vi "MHL Cases.vi"(8 "error in":errorcluster, 11 "Base Hardware in":refnum<class "Base Hardware.lvclass">) -> (0 "error out":errorcluster, 3 "Base Hardware out":refnum<class "Base Hardware.lvclass">)   [LabVIEW 2023, in "Abstract Hardware.lvlib" / "Base Hardware.lvclass"]
doc: "The base class Message Handling Loop cases of a Worker's QMH."
uses:
  Base Hardware.lvclass
  C:/Program Files/National Instruments/LabVIEW 2023/vi.lib/addons/_Workers/Library/Classes/Worker/Worker.lvclass
  <vilib>/addons/_Workers/Library/Classes/Worker/Worker.lvclass/Worker.ctl
  <vilib>/addons/_Workers/Library/Classes/Message/Message.lvclass/Message.ctl
  Initialization Data.ctl
  Response Cases.ctl
  <vilib>/addons/_Workers/Library/Case Label.ctl
  Settings.ctl
  Base Hardware.lvclass/Base Hardware.ctl
  rql_Read-Write Error.ctl
  rqp_Init.ctl
  rqp_Close.ctl
  rqp_Write.ctl
  rqp_Read.ctl
  rqp_REINIT.ctl
  rqp_Edit Polling.ctl
  rwr_Init With Reply.ctl
  rwr_Init With Reply Reply.ctl
  rqp_Update Internal Data.ctl
  rqp_Show Panel.ctl
  <vilib>/addons/_Workers/Library/Classes/Message/Priority.ctl
  <vilib>/Utility/error.llb/Error Cluster From Error Code.vi
  <vilib>/ErrorRing/Error Ring.xnode
  <vilib>/addons/_Workers/Library/Classes/Message Queue/Message Queue.lvclass
  <vilib>/addons/_Workers/Library/Classes/Worker/Worker.lvclass
  <vilib>/addons/_Workers/Library/Classes/Message/Message.lvclass
  Message Pump/Message Pump.lvclass
  <vilib>/addons/_Workers/Library/Workers.lvlib
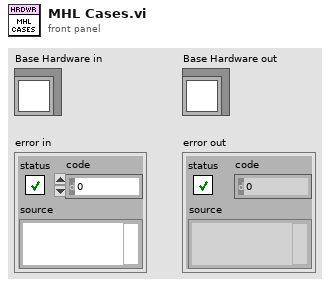
[diagram p1: front panel]
types:
  T1 = typedef "Workers.lvlib/Case Label.ctl" = string
  T2 = typedef "Abstract Hardware.lvlib/Base Hardware.lvclass/Initialization Data.ctl" = cluster{"Response Cases":T3, "Settings":T4}
  T3 = typedef "Abstract Hardware.lvlib/Base Hardware.lvclass/Response Cases.ctl" = cluster{"Placeholder - Can be deleted":string, "Get Data":T1, "Get Init Result":T1}
  T4 = typedef "Abstract Hardware.lvlib/Base Hardware.lvclass/Settings.ctl" = cluster{"Polling Period, ms":i64}
  T5 = typedef "Abstract Hardware.lvlib/Base Hardware.lvclass/rql_Read-Write Error.ctl" = cluster{"String":string}
  T6 = typedef "Abstract Hardware.lvlib/Base Hardware.lvclass/rqp_Init.ctl" = variant
  T7 = typedef "Abstract Hardware.lvlib/Base Hardware.lvclass/rqp_Close.ctl" = cluster{"String":string}
  T8 = typedef "Abstract Hardware.lvlib/Base Hardware.lvclass/rqp_Write.ctl" = variant
  T9 = typedef "Abstract Hardware.lvlib/Base Hardware.lvclass/rqp_Read.ctl" = cluster{"String":string}
  T10 = typedef "Abstract Hardware.lvlib/Base Hardware.lvclass/rqp_REINIT.ctl" = variant
  T11 = typedef "Abstract Hardware.lvlib/Base Hardware.lvclass/rqp_Edit Polling.ctl" = i64
  T12 = typedef "Abstract Hardware.lvlib/Base Hardware.lvclass/rwr_Init With Reply Reply.ctl" = cluster{"String":string}
  T13 = typedef "Abstract Hardware.lvlib/Base Hardware.lvclass/rwr_Init With Reply.ctl" = cluster{"String":string}
  T14 = typedef "Abstract Hardware.lvlib/Base Hardware.lvclass/rqp_Update Internal Data.ctl" = variant
  T15 = typedef "Abstract Hardware.lvlib/Base Hardware.lvclass/rqp_Show Panel.ctl" = cluster{"String":string}
  T16 = typedef "Workers.lvlib/Message.lvclass/Priority.ctl" = enum16{"Low", "Normal", "High"}
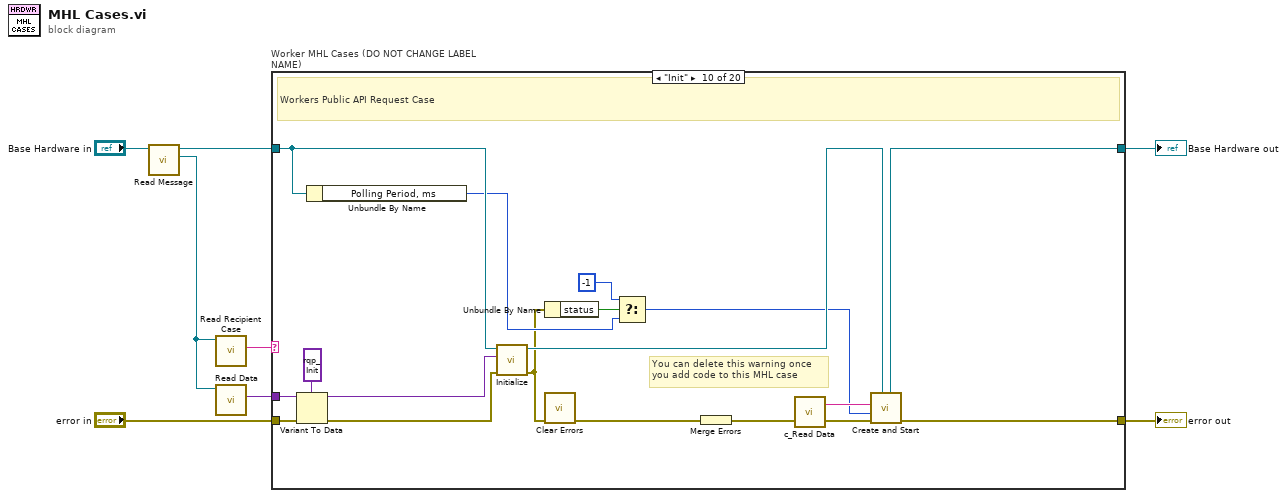
[diagram p0: block diagram]
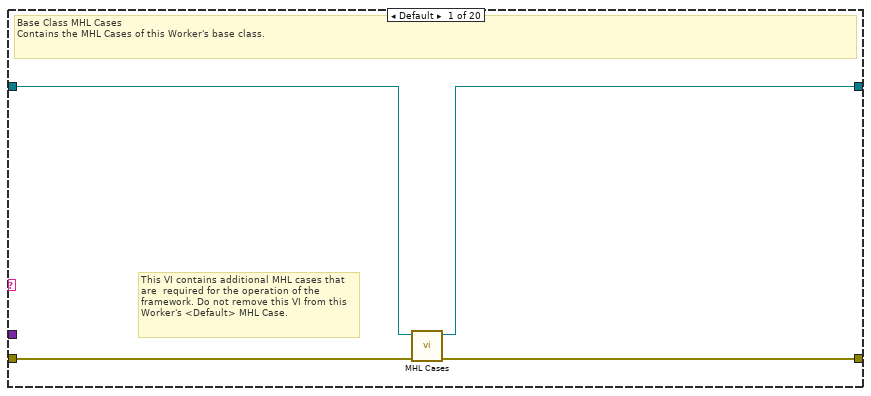
[diagram p2: hidden frame]
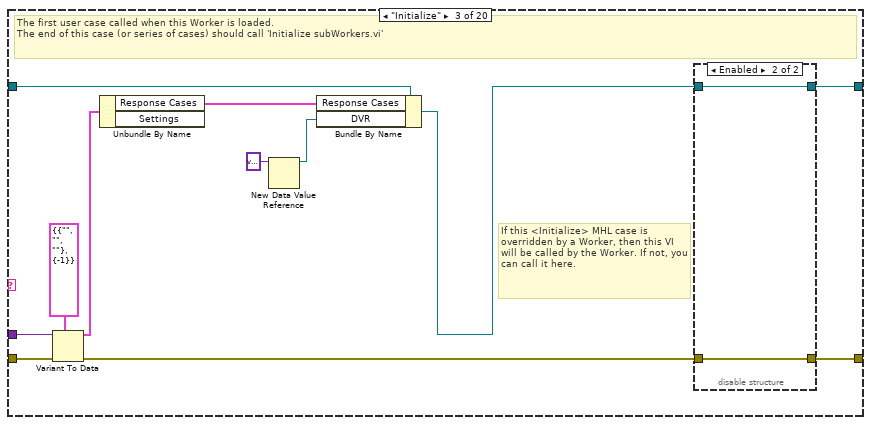
[diagram p4: hidden frame]
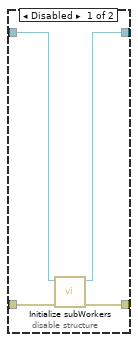
[diagram p5: hidden frame]
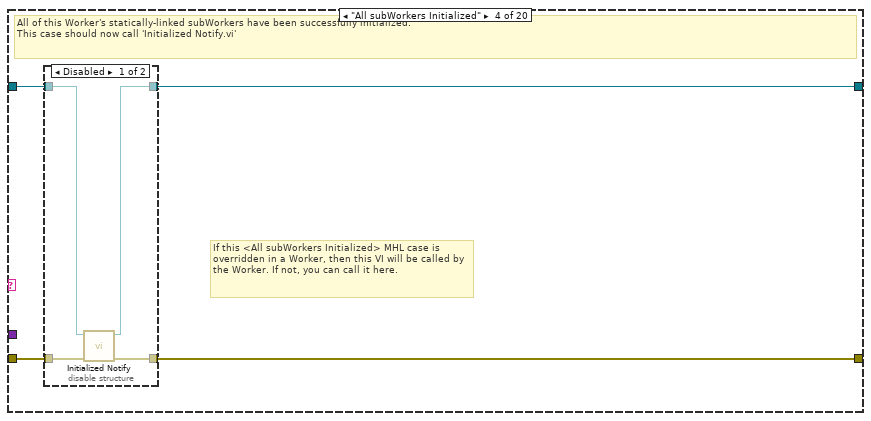
[diagram p6: hidden frame]
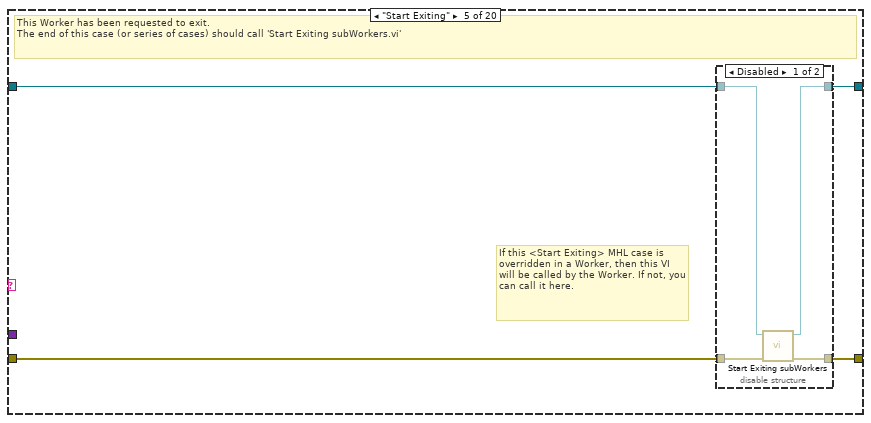
[diagram p8: hidden frame]
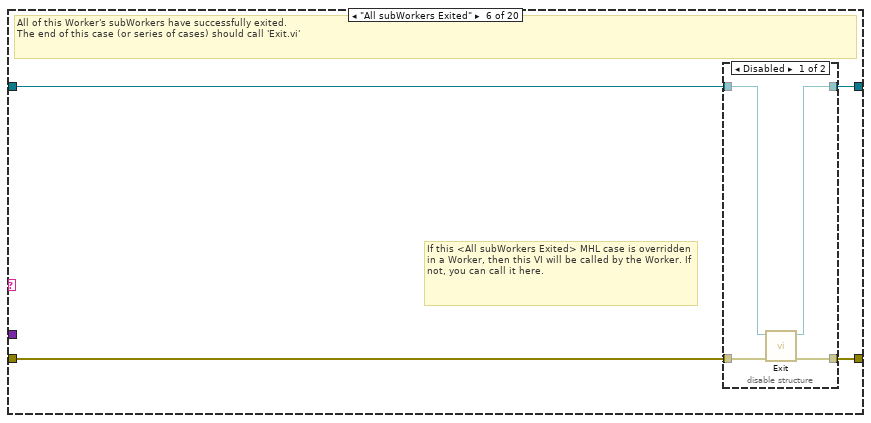
[diagram p10: hidden frame]
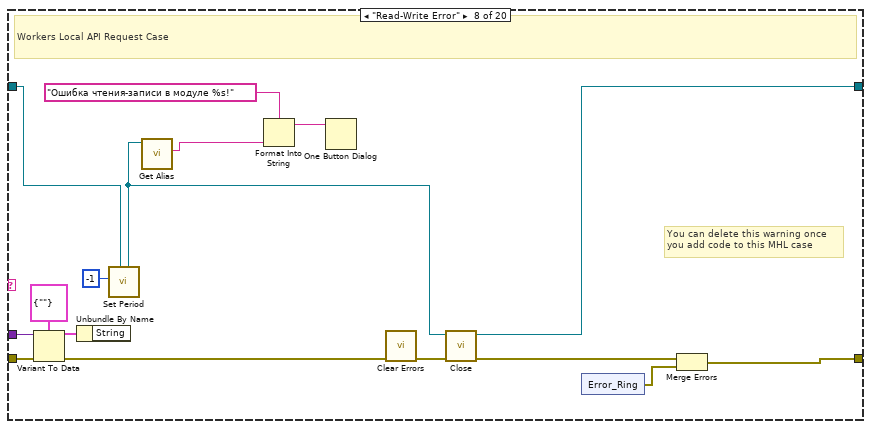
[diagram p13: hidden frame]
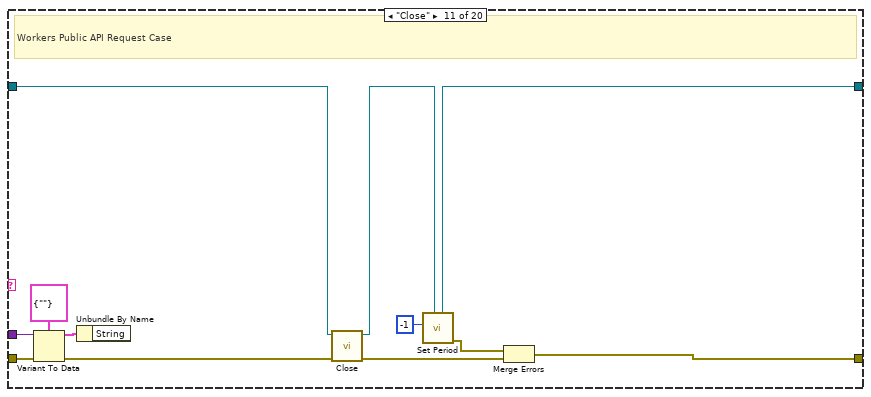
[diagram p15: hidden frame]
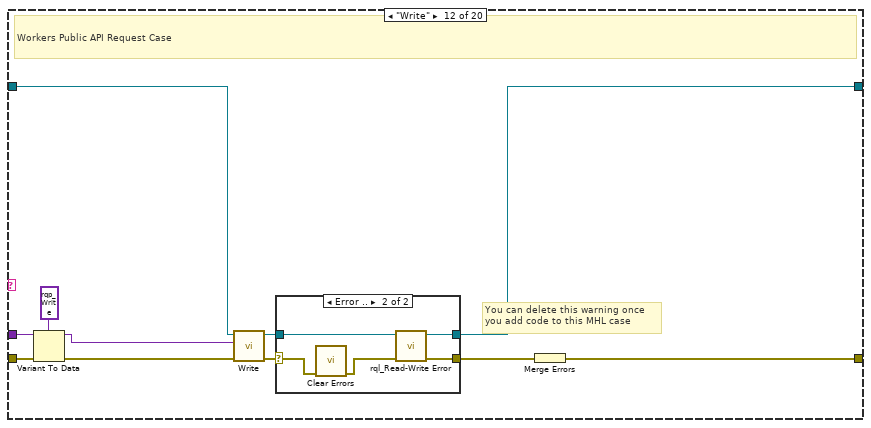
[diagram p16: hidden frame]
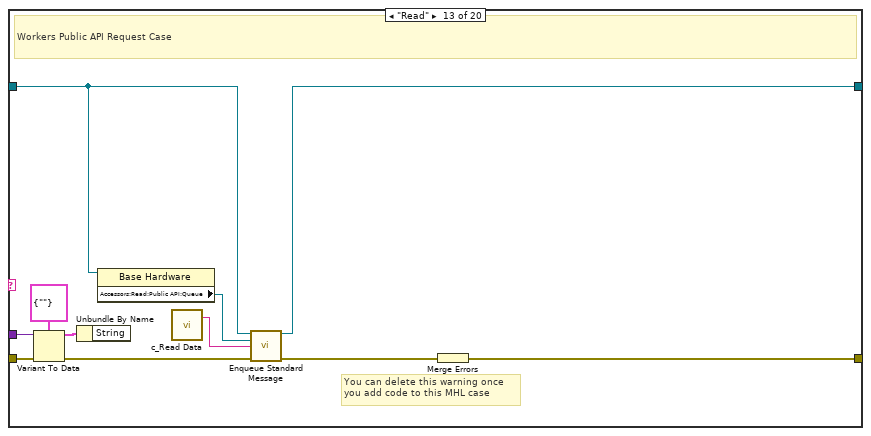
[diagram p18: hidden frame]
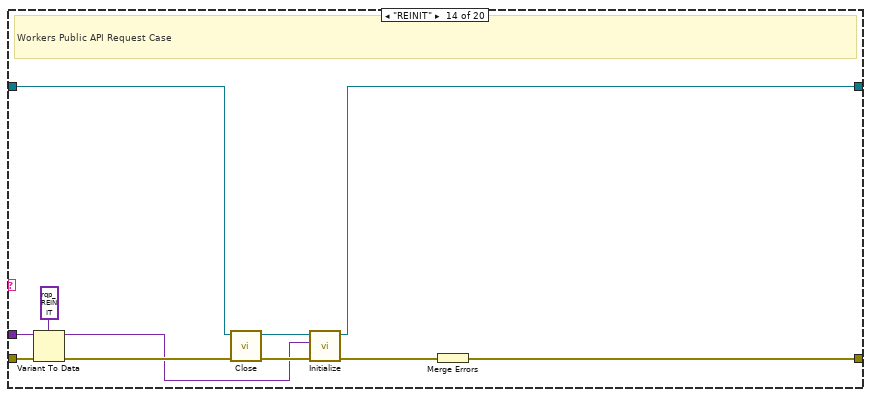
[diagram p19: hidden frame]
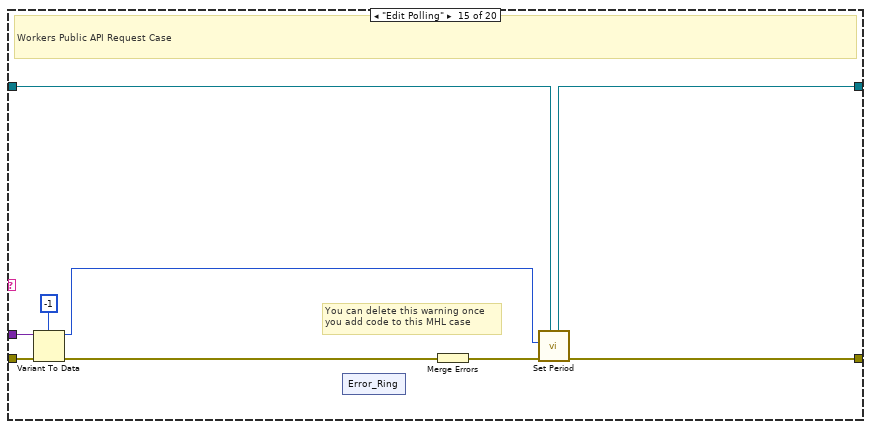
[diagram p20: hidden frame]
diagram:
  n1 = call <vilib>:"Read Message.vi"("Worker"="Base Hardware in") -> ("Message"=w3:refnum<class "Message.lvclass">, "dup Worker out"=w8:refnum<class "Base Hardware.lvclass">)  [unwired: 9 in]
  n2 = call <vilib>:"Read Recipient Case.vi"("Message"=w3) -> ("Recipient Case"=w7:T1)  [unwired: 9 in, 1 out]
  n3 = call <vilib>:"Read Data.vi"("Message"=w3) -> ("Data"=w1:variant)  [unwired: 9 in, 1 out]
  n4 = case "Worker MHL Cases (DO NOT CHANGE LABEL NAME)" shown="\"Init\"" w7 {
    tunnel: [w12 w14 w21 w33 w44 w55 w64 w76 w87 w88 w112 w121 w141 w153 w159 w176 w188 w205 w216 w219] -> w6
    tunnel: [w11 w13 w20 w35 w45 w53 w63 w71 w86 w100 w106 w119 w140 w146 w160 w175 w193 w200 w215 w220] -> w5
    tunnel: "error in" -> [w10 w14 w26 w34 w43 w56 w64 w80 w87 w104 w116 w127 w145 w156 w165 w181 w192 w209 w216 w221]
    tunnel: w8 -> [w9 w13 w17 w36 w46 w54 w63 w70 w86 w96 w109 w124 w136 w151 w161 w174 w193 w203 w215 w218]
    tunnel: w1 -> [_ _ w25 _ _ _ _ w78 _ w102 w114 w125 w143 w154 w162 w178 w189 w207 _ _]
    frame Default {
      # "This VI contains additional MHL cases that are  required for the operation of the framework. Do not remove this VI from this Worker's <Default> MHL Case."
      # "Base Class MHL Cases\nContains the MHL Cases of this Worker's base class."
      n5 = call-parent "MHL Cases.vi"("error in"=w10, "Worker in"=w9) -> ("error out"=w12:errorcluster, "Worker out"=w11:refnum<class "Base Hardware.lvclass">)  [unwired: 8 in]
    }
    frame "------------ FRAMEWORK CASES -----------" {
      # "Start of Workers Framework Cases"
    }
    frame "Initialize" {
      # "If this <Initialize> MHL case is overridden by a Worker, then this VI will be called by the Worker. If not, you can call it here."
      # "The first user case called when this Worker is loaded.\nThe end of this case (or series of cases) should call 'Initialize subWorkers.vi'"
      n6 = Variant To Data(error in=w26, type=T2 {"Response Cases"={"Placeholder - Can be deleted"="", "Get Data"="", "Get Init Result"=""}, "Settings"={"Polling Period, ms"=-1}} ("Initialization Data"), Variant=w25) -> (data=w24:T2, error out=w15:errorcluster)
      n7 = Unbundle By Name(w24) -> ("Response Cases"=w23:T3)  [unwired: 1 out]
      n8 = New Data Value Reference(data value=variant) -> (data value reference=w18:refnum<data-value>)  [unwired: 1 in, 1 out]
      n9 = Bundle By Name(cluster=w17, "Response Cases"=w23, "DVR"=w18) -> (w16:refnum<class "Base Hardware.lvclass">)
      n10 = disable-structure shown="Enabled" {
        disable-tunnel: w15 -> [w30 w31]
        disable-tunnel: [w29 w31] -> w21
        disable-tunnel: w16 -> [w28 w32]
        disable-tunnel: [w27 w32] -> w20
        frame Disabled {
          n11 = call-dynamic "Initialize subWorkers.vi"("error in"=w30, "Base Hardware"=w28) -> ("error out"=w29:errorcluster, "dup Base Hardware out"=w27:refnum<class "Base Hardware.lvclass">)  [unwired: 8 in]
        }
        frame Enabled {
        }
      }
    }
    frame "All subWorkers Initialized" {
      # "If this <All subWorkers Initialized> MHL case is overridden in a Worker, then this VI will be called by the Worker. If not, you can call it here."
      # "All of this Worker's statically-linked subWorkers have been successfully initialized.\nThis case should now call 'Initialized Notify.vi'"
      n12 = disable-structure shown="Disabled" {
        disable-tunnel: w36 -> [w40 w42]
        disable-tunnel: [w39 w42] -> w35
        disable-tunnel: w34 -> [w38 w41]
        disable-tunnel: [w37 w41] -> w33
        frame Disabled {
          n13 = call-dynamic "Initialized Notify.vi"("error in"=w38, "Worker"=w40) -> ("error out"=w37:errorcluster, "dup Worker out"=w39:refnum<class "Base Hardware.lvclass">)  [unwired: 8 in]
        }
        frame Enabled {
        }
      }
    }
    frame "Start Exiting" {
      # "If this <Start Exiting> MHL case is overridden in a Worker, then this VI will be called by the Worker. If not, you can call it here."
      # "This Worker has been requested to exit. \nThe end of this case (or series of cases) should call 'Start Exiting subWorkers.vi'"
      n14 = disable-structure shown="Disabled" {
        disable-tunnel: w46 -> [w50 w52]
        disable-tunnel: [w49 w52] -> w45
        disable-tunnel: [w48 w51] -> w44
        disable-tunnel: w43 -> [w47 w51]
        frame Disabled {
          n15 = call-dynamic "Start Exiting subWorkers.vi"("error_in"=w47, "Worker"=w50) -> ("error out"=w48:errorcluster, "dup Worker out"=w49:refnum<class "Base Hardware.lvclass">)  [unwired: 8 in]
        }
        frame Enabled {
        }
      }
    }
    frame "All subWorkers Exited" {
      # "If this <All subWorkers Exited> MHL case is overridden in a Worker, then this VI will be called by the Worker. If not, you can call it here."
      # "All of this Worker's subWorkers have successfully exited. \nThe end of this case (or series of cases) should call 'Exit.vi'"
      n16 = disable-structure shown="Disabled" {
        disable-tunnel: w56 -> [w60 w61]
        disable-tunnel: [w59 w61] -> w55
        disable-tunnel: w54 -> [w58 w62]
        disable-tunnel: [w57 w62] -> w53
        frame Disabled {
          n17 = call-dynamic "Exit.vi"("error_in"=w60, "Worker"=w58) -> ("error out"=w59:errorcluster, "dup Worker out"=w57:refnum<class "Base Hardware.lvclass">)  [unwired: 8 in]
        }
        frame Enabled {
        }
      }
    }
    frame "------------- LOCAL API CASES -------------" {
      # "Start of Workers Local API Cases"
    }
    frame "Read-Write Error" {
      # "You can delete this warning once\nyou add code to this MHL case"
      # "Workers Local API Request Case"
      n18 = Variant To Data(error in=w80, type=T5 {"String"=""} ("Data"), Variant=w78) -> (data=w77:T5, error out=w66:errorcluster)
      n19 = Unbundle By Name(w77) -> ()  [unwired: 1 out]
      n20 = call "Set Period.vi"("Caller"=w70, "Period (ms)"=-1) -> ("dup Caller out"=w69:refnum<class "Base Hardware.lvclass">)  [unwired: 8 in, 1 out]
      n21 = call-dynamic "Get Alias.vi"("Worker_"=w69) -> ("Alias"=w67:string)  [unwired: 8 in, 2 out]
      n22 = Format Into String(format string="Ошибка чтения-записи в модуле %s!", w67) -> (resulting string=w65:string)  [unwired: 2 in, 1 out]
      n23 = One Button Dialog(message=w65) -> ()  [unwired: 1 in, 1 out]
      n24 = call <vilib>:"Clear Errors.vi"("error in (no error)"=w66) -> ("error out"=w73:errorcluster)  [unwired: 5 in, 1 out]
      n25 = call-dynamic "Close.vi"("error in (no error)"=w73, "Base Hardware in"=w69) -> ("error out"=w72:errorcluster, "Base Hardware out"=w71:refnum<class "Base Hardware.lvclass">)  [unwired: 8 in]
      n26 = xnode ("Error_Ring")() -> ("error out"=w75:errorcluster)
      n27 = Merge Errors(w72, w75) -> (w76:errorcluster)
    }
    frame "------------- PUBLIC API CASES -------------" {
      # "Start of Workers Public API Cases"
    }
    frame "Init" {
      # "You can delete this warning once\nyou add code to this MHL case"
      # "Workers Public API Request Case"
      n28 = Variant To Data(error in=w104, type=T6 variant(string "") ("Data"), Variant=w102) -> (data=w95:T6, error out=w97:errorcluster)
      n29 = Unbundle By Name(w96) -> ("Polling Period, ms"=w93:i64)
      n30 = call-dynamic "Initialize.vi"("error in (no error)"=w97, "Settings"=w95, "Base Hardware in"=w96) -> ("error out"=w89:errorcluster, "Base Hardware out"=w98:refnum<class "Base Hardware.lvclass">)  [unwired: 7 in]
      n31 = Unbundle By Name(w89) -> ("status"=w94:bool)
      n32 = call <vilib>:"Clear Errors.vi"("error in (no error)"=w89) -> ("error out"=w90:errorcluster)  [unwired: 5 in, 1 out]
      n33 = Select(t=i64 -1, s=w94, f=w93) -> (s? t:f=w91:i64)
      n34 = Merge Errors(w90) -> (w99:errorcluster)
      n35 = call "c_Read Data.vi"() -> ("Case Label"=w101:T1)  [unwired: 1 in]
      n36 = call "Create and Start.vi"("Caller"=w98, "error in (no error)"=w99, "Period (ms)"=w91, "Time Elapsed Response Case (Case Label)"=w101) -> ("error out"=w88:errorcluster, "dup Caller out"=w100:refnum<class "Base Hardware.lvclass">)  [unwired: 5 in, 1 out]
    }
    frame "Close" {
      # "Workers Public API Request Case"
      n37 = Variant To Data(error in=w116, type=T7 {"String"=""} ("Data"), Variant=w114) -> (data=w113:T7, error out=w111:errorcluster)
      n38 = Unbundle By Name(w113) -> ()  [unwired: 1 out]
      n39 = call-dynamic "Close.vi"("error in (no error)"=w111, "Base Hardware in"=w109) -> ("error out"=w110:errorcluster, "Base Hardware out"=w107:refnum<class "Base Hardware.lvclass">)  [unwired: 8 in]
      n40 = call "Set Period.vi"("Caller"=w107, "Period (ms)"=-1) -> ("error out"=w108:errorcluster, "dup Caller out"=w106:refnum<class "Base Hardware.lvclass">)  [unwired: 8 in]
      n41 = Merge Errors(w108, w110) -> (w112:errorcluster)
    }
    frame "Write" {
      # "You can delete this warning once\nyou add code to this MHL case"
      # "Workers Public API Request Case"
      n42 = Variant To Data(error in=w127, type=T8 variant(string "") ("Data"), Variant=w125) -> (data=w122:T8, error out=w123:errorcluster)
      n43 = call-dynamic "Write.vi"("error in (no error)"=w123, "Write Data"=w122, "Base Hardware in"=w124) -> ("error out"=w117:errorcluster, "Base Hardware out"=w118:refnum<class "Base Hardware.lvclass">)  [unwired: 7 in]
      n44 = case shown="Error .." w117 {
        selector: w117 -> [w128 w131]
        tunnel: [w128 w132] -> w120
        tunnel: [w129 w133] -> w119
        tunnel: w118 -> [w129 w134]
        frame No Error {
        }
        frame Error {
          n45 = call <vilib>:"Clear Errors.vi"("error in (no error)"=w131) -> ("error out"=w130:errorcluster)  [unwired: 5 in, 1 out]
          n46 = call "rql_Read-Write Error.vi"("error in"=w130, "Base Hardware in"=w134) -> ("error out"=w132:errorcluster, "dup Base Hardware out"=w133:refnum<class "Base Hardware.lvclass">)  [unwired: 8 in]
        }
      }
      n47 = Merge Errors(w120) -> (w121:errorcluster)
    }
    frame "Read" {
      # "You can delete this warning once\nyou add code to this MHL case"
      # "Workers Public API Request Case"
      n48 = Variant To Data(error in=w145, type=T9 {"String"=""} ("Data"), Variant=w143) -> (data=w142:T9, error out=w139:errorcluster)
      n49 = Unbundle By Name(w142) -> ()  [unwired: 1 out]
      n50 = property class="Base Hardware"(reference=w136) -> ("Accessors:Read:Public API:Queue"=w135:refnum<class "Message Queue.lvclass">)  [unwired: 1 in, 2 out]
      n51 = call "c_Read Data.vi"() -> ("Case Label"=w137:T1)  [unwired: 1 in]
      n52 = call-dynamic "Enqueue Standard Message.vi"("Worker"=w136, "Message Queue"=w135, "Case Label"=w137, "error in (no error)"=w139) -> ("dup Worker out"=w140:refnum<class "Base Hardware.lvclass">, "error out"=w138:errorcluster)  [unwired: 10 in]
      n53 = Merge Errors(w138) -> (w141:errorcluster)
    }
    frame "REINIT" {
      # "Workers Public API Request Case"
      n54 = Variant To Data(error in=w156, type=T10 variant(string "") ("Data"), Variant=w154) -> (data=w147:T10, error out=w152:errorcluster)
      n55 = call-dynamic "Close.vi"("error in (no error)"=w152, "Base Hardware in"=w151) -> ("error out"=w150:errorcluster, "Base Hardware out"=w148:refnum<class "Base Hardware.lvclass">)  [unwired: 8 in]
      n56 = call-dynamic "Initialize.vi"("error in (no error)"=w150, "Settings"=w147, "Base Hardware in"=w148) -> ("error out"=w149:errorcluster, "Base Hardware out"=w146:refnum<class "Base Hardware.lvclass">)  [unwired: 7 in]
      n57 = Merge Errors(w149) -> (w153:errorcluster)
    }
    frame "Edit Polling" {
      # "You can delete this warning once\nyou add code to this MHL case"
      # "Workers Public API Request Case"
      n58 = Variant To Data(error in=w165, type=T11 -1 ("Data"), Variant=w162) -> (data=w157:T11, error out=w164:errorcluster)
      n59 = xnode ("Error_Ring")() -> ()  [unwired: 1 out]
      n60 = Merge Errors(w164) -> (w158:errorcluster)
      n61 = call "Set Period.vi"("Caller"=w161, "error in"=w158, "Period (ms)"=w157) -> ("error out"=w159:errorcluster, "dup Caller out"=w160:refnum<class "Base Hardware.lvclass">)  [unwired: 7 in]
    }
    frame "Init With Reply" {
      # "You can delete this warning once\nyou add code to this MHL case"
      # "Workers Public API Request w/Reply Case"
      n62 = Variant To Data(error in=w181, type=T13 {"String"=""} ("Data"), Variant=w178) -> (data=w177:T13, error out=w180:errorcluster)
      n63 = Unbundle By Name(w177) -> ()  [unwired: 1 out]
      n64 = xnode ("Error_Ring")() -> ("error out"=w171:errorcluster)
      n65 = Merge Errors(w180, w171) -> (w172:errorcluster)
      n66 = call-dynamic "Callback Easy Reply.vi"("error in"=w172, "Data"=T12 {"String"=""} ("Reply Data"), "Worker"=w174) -> ("error out"=w176:errorcluster, "dup Worker out"=w175:refnum<class "Base Hardware.lvclass">)  [unwired: 7 in]
    }
    frame "Update Internal Data" {
      # "You can delete this warning once\nyou add code to this MHL case"
      # "Workers Public API Request Case"
      n67 = Variant To Data(error in=w192, type=T14 variant(string "") ("Data"), Variant=w189) -> (error out=w191:errorcluster)  [unwired: 1 out]
      n68 = xnode ("Error_Ring")() -> ("error out"=w187:errorcluster)
      n69 = Merge Errors(w191, w187) -> (w188:errorcluster)
    }
    frame "Show Panel" {
      # "You can delete this warning once\nyou add code to this MHL case"
      # "Workers Public API Request Case"
      n70 = Variant To Data(error in=w209, type=T15 {"String"=""} ("Data"), Variant=w207) -> (data=w206:T15, error out=w202:errorcluster)
      n71 = Unbundle By Name(w206) -> ()  [unwired: 1 out]
      n72 = call-dynamic "Get MainVI Ref.vi"("error in (no error)"=w202, "Worker_"=w203) -> ("error out"=w201:errorcluster, "MainVI Ref"=w199:refnum<vi>, "dup Worker_out"=w200:refnum<class "Base Hardware.lvclass">)  [unwired: 7 in]
      n73 = xnode ("Error_Ring")() -> ("error out"=w204:errorcluster)
      n74 = invoke class="VI" method="FP.Open"(reference=w199) -> ()  [unwired: 4 in, 5 out]
      n75 = Merge Errors(w201, w204) -> (w205:errorcluster)
    }
    frame "------------- RESPONSE CASES --------------" {
      # "Start of Workers Response Cases"
    }
    frame "Read Data" {
      # "This case receives a Response message from a subWorker"
      n76 = Unbundle By Name(w218) -> ("Use?"=w217:bool)
      n77 = case shown="True" w217 {
        tunnel: w221 -> [w222 w239]
        tunnel: [w223 w233] -> w220
        tunnel: [w222 w231] -> w219
        tunnel: w218 -> [w223 w224]
        frame False {
        }
        frame True {
          n78 = Unbundle By Name(w224) -> ("DVR"=w237:refnum<data-value>)
          n79 = call-dynamic "Read.vi"("error in (no error)"=w239, "Base Hardware in"=w224) -> ("error out"=w230:errorcluster, "Read Data"=w226:variant, "Base Hardware out"=w227:refnum<class "Base Hardware.lvclass">)  [unwired: 7 in]
          n80 = case shown="Error .." w230 {
            selector: w230 -> [w240 w244]
            tunnel: [w240 w245] -> w229
            tunnel: [w241 w246] -> w228
            tunnel: w227 -> [w241 w242]
            frame No Error {
            }
            frame Error {
              n81 = call <vilib>:"Clear Errors.vi"("error in (no error)"=w244) -> ("error out"=w243:errorcluster)  [unwired: 5 in, 1 out]
              n82 = call "rql_Read-Write Error.vi"("error in"=w243, "Base Hardware in"=w242) -> ("error out"=w245:errorcluster, "dup Base Hardware out"=w246:refnum<class "Base Hardware.lvclass">)  [unwired: 8 in]
            }
          }
          n83 = in-place {
            in-place-border: w226 -> [w247]
            n84 = in-place-dvr #1(w237) -> ()  [unwired: 2 out]
            n85 = in-place-dvr #1(w247) -> (w235:refnum<data-value>)  [unwired: 1 out]
          }
          n86 = call "rsp_Get Data.vi"("error in"=w229, "Data in"=w226, "Base Hardware in"=w228) -> ("error out"=w238:errorcluster, "dup Base Hardware out"=w236:refnum<class "Base Hardware.lvclass">)  [unwired: 7 in]
          n87 = Bundle By Name(cluster=w236, "DVR"=w235) -> (w234:refnum<class "Base Hardware.lvclass">)
          n88 = Merge Errors(w238) -> (w232:errorcluster)
          n89 = call "rqp_Update Internal Data.vi"("Message Priority"=Priority."Low", "error in"=w232, "Data in"=w226, "Base Hardware in"=w234) -> ("error out"=w231:errorcluster, "dup Base Hardware out"=w233:refnum<class "Base Hardware.lvclass">)  [unwired: 5 in, 1 out]
        }
      }
    }
  }
  "Base Hardware out" <- w5
  "error out" <- w6
